vi "CaptureImageAtPosition(Sync).vi"(6 "timeout in ms (5000)":i32=5000, 8 "error in (no error)":errorcluster, 10 "Coords":T1, 11 "Microscope":refnum<class "Microscope.lvclass">) -> (0 "error out":errorcluster, 2 "buffer":i32, 3 "Microscope out":refnum<class "Microscope.lvclass">)   [LabVIEW 2013, in "Microscope.lvclass"]
doc: "---------------------------------------------------------------\nJKI State Machine Objects™\nhttp://jki.net/state-machine-objects/\nCopyright (C) 2005-2015, JKI <info@jki.net>\nALL RIGHTS RESERVEDJKI State Machine Objects (SMO) 1.0.0.4\nJKI - JKI\nCopyright (c) 2015, JKI"
uses:
  Microscope.lvclass
  XYStage/Typedefs/(real)Coords--Cluster.ctl
  XYStage/XYStage.lvclass
panel:
  # "For instructions on how to use the JKI State Machine Objects, examples and video tutorials, visit:\nhttp://jki.net/state-machine-objects/\n\nJKI State Machine Objects™\nhttp://jki.net/state-machine-objects/\nCopyright (C) 2005-2015, JKI <info@jki.net>\nALL RIGHTS RESERVED"
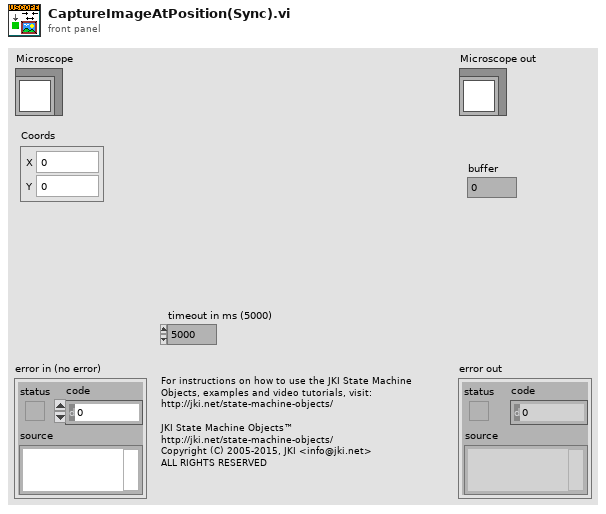
[diagram p1: front panel]
types:
  T1 = typedef "XYStage.lvclass/(real)Coords--Cluster.ctl" = cluster{"X":dbl, "Y":dbl}
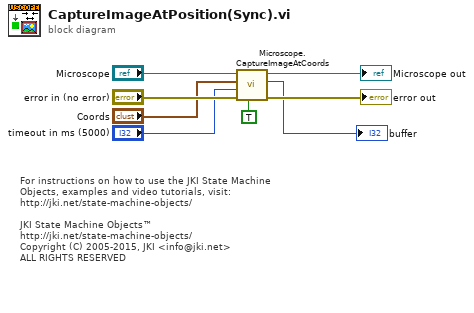
[diagram p0: block diagram]
diagram:
  # "For instructions on how to use the JKI State Machine Objects, examples and video tutorials, visit:\nhttp://jki.net/state-machine-objects/\n\nJKI State Machine Objects™\nhttp://jki.net/state-machine-objects/\nCopyright (C) 2005-2015, JKI <info@jki.net>\nALL RIGHTS RESERVED"
  n1 = call "Microscope.CaptureImageAtCoords.vi"("Move?"=TRUE, "error in (no error)"="error in (no error)", "timeout (5000 ms)"="timeout in ms (5000)", "Coords"="Coords", "Microscope"="Microscope") -> ("error out"=→"error out":errorcluster, "buffer"=→"buffer":i32, "Microscope out"=→"Microscope out":refnum<class "Microscope.lvclass">)  [unwired: 3 in, 1 out]
